vi "Request Data.vi"(6 "Qualifier":string, 8 "error in":errorcluster, 9 "notifier":refnum<notifier>, 10 "Data to Send":string, 11 "AnalogInput in":refnum<class "AnalogInput.lvclass">) -> (0 "error out":errorcluster, 3 "AnalogInput out":refnum<class "AnalogInput.lvclass">)   [LabVIEW 2019, in "AnalogInput.lvlib" / "AnalogInput.lvclass"]
doc: "Data to Send is a required input that describes the measurement or query function to be performed\nQualifier is a secondary variable used in the event that specificity must be provided to the query function\n****Note****\nIf further specificity is required, the qualifier must be used in a comma delimited format to increase the overall variable count. Additional specificity must be provided by the child class and interpreted by the automated call.\n\nnotifier is a single variant notifier in which the instrument will send the data notification to the automated tool."
uses:
  Library/AnalogInput.lvclass
  C:/Users/Public/Documents/Development/builds/Instruments/Instruments.lvlibp/Library/Instruments.lvclass
  Library/AnalogInput.lvclass/AnalogInput.ctl
  Accessors/GUI/Read Snapshot_Timeout.vi
  builds/Instruments/Instruments.lvlibp/Private/Accessors/Read Poll(ms).vi
  builds/Instruments/Instruments.lvlibp/Accessors/Read Measured.vi
  builds/Instruments/Instruments.lvlibp/Accessors/Read Snapshot.vi
  builds/Instruments/Instruments.lvlibp/Private/Polymorphic/Special/Event from String.vi
  builds/Instruments/Instruments.lvlibp/Accessors/Command with Logging.vi
  builds/Instruments/Instruments.lvlibp/Library/Instruments.lvclass
  builds/Instruments/Instruments.lvlibp
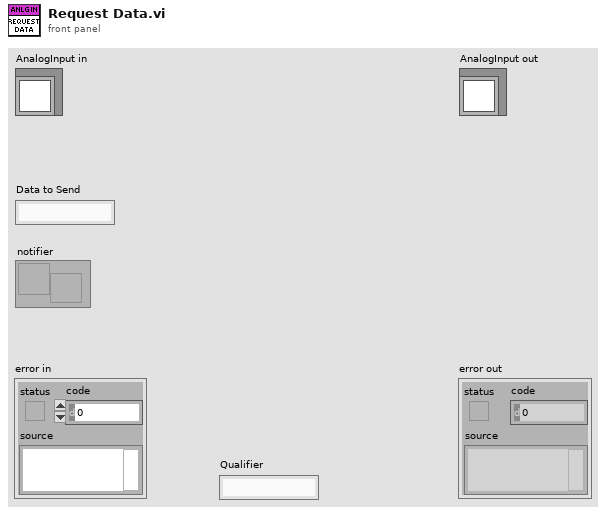
[diagram p1: front panel]
types:
  T1 = cluster{"Timestamp":timestamp, "Description":string, "Data":string}
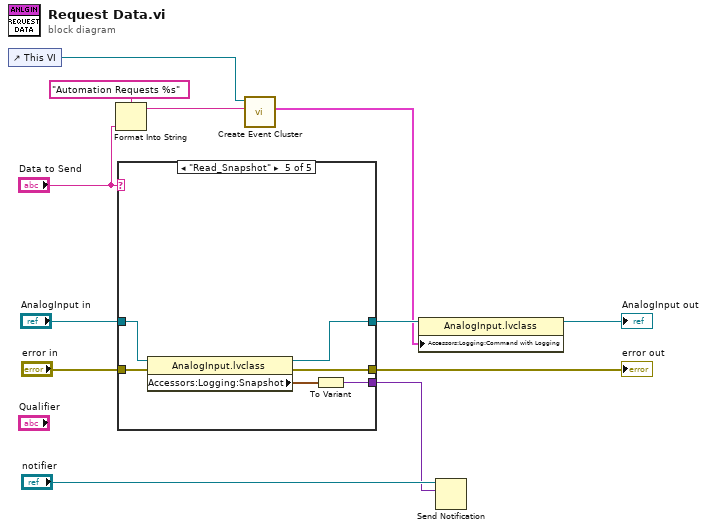
[diagram p0: block diagram]
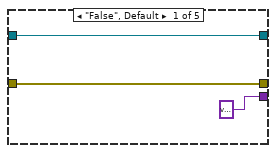
[diagram p2: hidden frame]
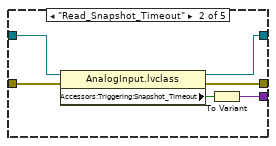
[diagram p3: hidden frame]
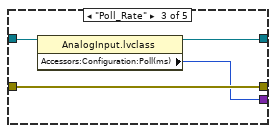
[diagram p4: hidden frame]
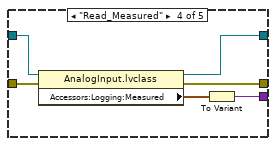
[diagram p5: hidden frame]
diagram:
  n1 = control-ref of="This VI"() -> (w4:refnum<vi>)
  n2 = Format Into String(format string="Automation Requests %s", "Data to Send") -> (resulting string=w5:string)  [unwired: 2 in, 1 out]
  n3 = case shown="\"Read_Snapshot\"" "Data to Send" {
    tunnel: "AnalogInput in" -> [w15 w21 w25 w31 w37]
    tunnel: "error in" -> [w14 w20 w23 w29 w35]
    tunnel: [w15 w19 w24 w30 w36] -> w3
    tunnel: [w14 w18 w23 w28 w34] -> w9
    tunnel: [variant w16 w22 w27 w33] -> w8
    frame "False", Default {
    }
    frame "Read_Snapshot_Timeout" {
      n4 = property class="AnalogInput.lvclass"(reference=w21, error in=w20) -> (reference out=w19:refnum<class "AnalogInput.lvclass">, error out=w18:errorcluster, "Accessors:Triggering:Snapshot_Timeout"=w17:bool)
      n5 = To Variant(anything=w17) -> (Variant=w16:variant)
    }
    frame "Poll_Rate" {
      n6 = property class="AnalogInput.lvclass"(reference=w25) -> (reference out=w24:refnum<class "AnalogInput.lvclass">, "Accessors:Configuration:Poll(ms)"=w22:u32)  [unwired: 1 in, 1 out]
    }
    frame "Read_Measured" {
      n7 = property class="AnalogInput.lvclass"(reference=w31, error in=w29) -> (reference out=w30:refnum<class "AnalogInput.lvclass">, error out=w28:errorcluster, "Accessors:Logging:Measured"=w26:waveform(dbl)[])
      n8 = To Variant(anything=w26) -> (Variant=w27:variant)
    }
    frame "Read_Snapshot" {
      n9 = property class="AnalogInput.lvclass"(reference=w37, error in=w35) -> (reference out=w36:refnum<class "AnalogInput.lvclass">, error out=w34:errorcluster, "Accessors:Logging:Snapshot"=w32:waveform(dbl)[])
      n10 = To Variant(anything=w32) -> (Variant=w33:variant)
    }
  }
  "error out" <- w9
  n11 = call-poly "Create Event Cluster.vi"("Value"=w5, "VI Refnum"=w4) -> ("Event Data"=w1:T1)  [unwired: 9 in]
  n12 = property class="AnalogInput.lvclass"(reference=w3, "Accessors:Logging:Command with Logging"=w1) -> (reference out=→"AnalogInput out":refnum<class "AnalogInput.lvclass">)  [unwired: 1 in, 1 out]
  n13 = Send Notification(notification=w8, notifier="notifier") -> ()  [unwired: 1 in, 2 out]
